vi "FdxCmdTxVLWriteCvi.vi"(8 "error in":errorcluster, 9 "TxVLWriteIn":T1, 11 "InstrumentHandle":u32) -> (0 "error out":errorcluster, 1 "BytesWritten":u32, 3 "InstrumentHandle":u32)   [LabVIEW 2020, in "AIM664LV.lvlib"]
doc: "This function is used to write data directly to a virtual link buffer. The Virtual link has to be defined using function AiFdxCmdTxCreateVL."
uses:
  AIM664LV.lvlib
  AFDX_LibraryAdmin/FdxGlobalDllPath.vi
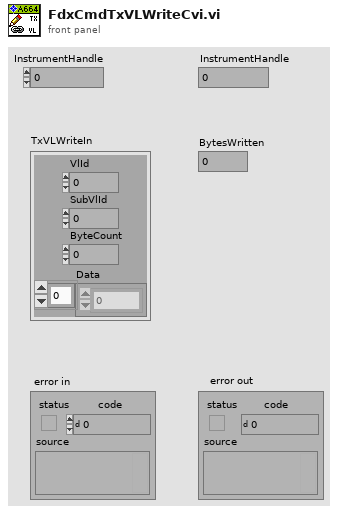
[diagram p1: front panel]
types:
  T1 = cluster{"VlId":u32, "SubVlId":u32, "ByteCount":u32, "Data":u8[]}
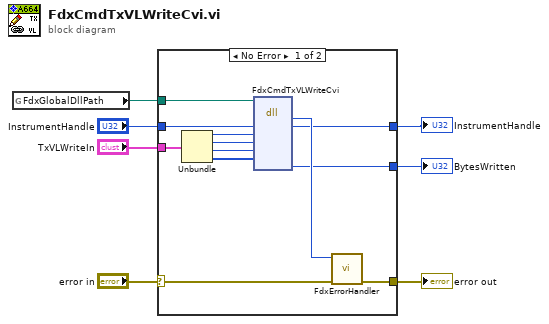
[diagram p0: block diagram]
diagram:
  n1 = global read "FdxGlobalDllPath.vi" "FdxGlobalDllPath"() -> (w5:path)
  n2 = case shown="No Error" "error in" {
    selector: "error in" -> [w18 w21]
    tunnel: [w19 w21] -> w7
    tunnel: w5 -> [w12 _]
    tunnel: "InstrumentHandle" -> [w11 w20]
    tunnel: [w10 w20] -> w3
    tunnel: [w9 _] -> w2
    tunnel: "TxVLWriteIn" -> [w8 _]
    frame No Error {
      n3 = Unbundle(w8) -> ("VlId"=w16:u32, "SubVlId"=w15:u32, "ByteCount"=w14:u32, "Data"=w13:u8[])
      n4 = dll-call lib="aim_fdx.19.dll" fn="FdxCmdTxVLWriteCvi"(path in=w12, "InstrumentHandle"=w11, "VlId"=w16, "SubVlId"=w15, "ByteCount"=w14, "Data"=w13) -> ("status"=w17:i32, "InstrumentHandle"=w10:u32, "BytesWritten"=w9:u32)  [unwired: 6 in, 3 out]
      n5 = call "FdxErrorHandler.vi"("error in"=w18, "AIM Error"=w17) -> ("error out"=w19:errorcluster)  [unwired: 9 in]
    }
    frame Error {
    }
  }
  "error out" <- w7
  "InstrumentHandle" <- w3
  "BytesWritten" <- w2
